vi "Format Site Specific Query (SubVI).vi"(1 "Table":string, 2 "Site":string) -> (0 "Query":string)   [LabVIEW 2015]
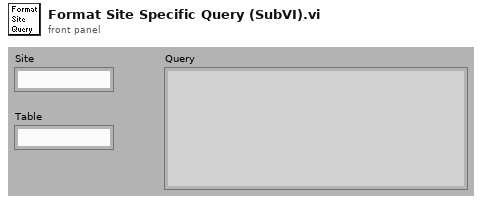
[diagram p1: front panel]
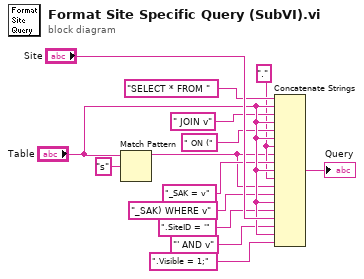
[diagram p0: block diagram]
diagram:
  w6 = "." ("SQL query")
  n1 = Match Pattern(string="Table", regular expression="s") -> (before substring=w5:string)  [unwired: 4 out]
  n2 = Concatenate Strings("SELECT * FROM " ("SQL query"), "Table", " JOIN v" ("SQL query"), "Table", " ON (" ("SQL query"), "Table", w6, w5, "_SAK = v" ("SQL query"), "Table", w6, w5, "_SAK) WHERE v" ("SQL query"), "Table", ".SiteID = '" ("SQL query"), "Site", "' AND v" ("SQL query"), "Table", ".Visible = 1;" ("SQL query")) -> (→"Query":string)
